vi "boolean mechanical action tests.vi"() -> ()   [LabVIEW 2021, in "Test VIs.lvclass"]
uses:
  Main VIs/Test VIs/Test VIs.lvclass
panel:
  out "Radio Buttons 2":enum32{"Radio Selection 1", "Radio Selection 2"}(radio)
  in  "Radio Buttons":enum32{"Radio Selection 1", "Radio Selection 2"}(radio)
  in  "stop":bool
  out "Boolean 3":bool
  out "Boolean 2":bool
  out "Boolean":bool
  out "Latch Until Released":string
  out "Latch When Released":string
  out "Latch When Pressed":string
  out "Switch Until Released":string
  out "Switch When Released":string
  out "Switch When Pressed":string
  in  "Latch Until Released":bool
  in  "Latch When Released":bool
  in  "Latch When Pressed":bool
  in  "Switch Until Released":bool
  in  "Switch When Released":bool
  in  "Switch When Pressed":bool
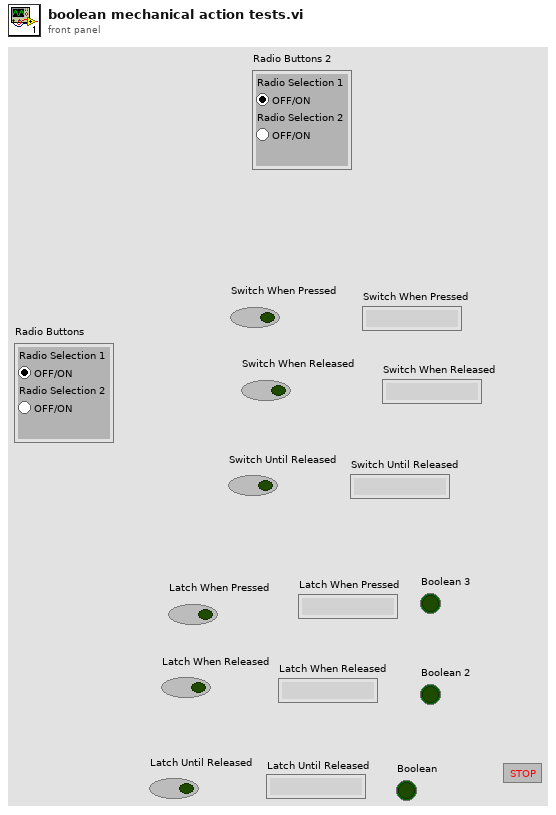
[diagram p1: front panel]
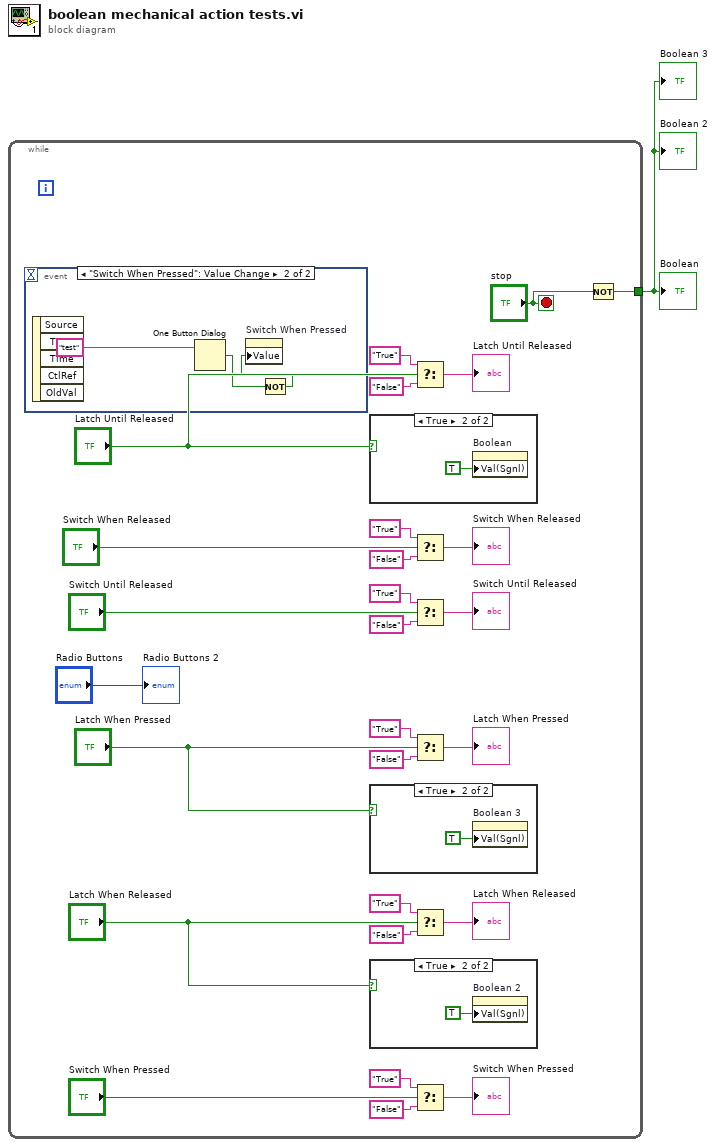
[diagram p0: block diagram]
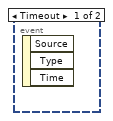
[diagram p2: hidden frame]
diagram:
  n1 = while {
    tunnel: [w4] -> w1
    stop <- "stop" stop-if-true
    n2 = event shown="[1] \"Switch When Pressed\": Value Change" {
      selector: _ -> [_ _]
      dyn-events: _ -> [_ _]
      timeout: _ -> [_ _]
      event Timeout {
        n3 = event-data() -> ()  [unwired: 1 in, 3 out]
      }
      event "Switch When Pressed": Value Change {
        n4 = event-data() -> ()  [unwired: 1 in, 5 out]
        n5 = One Button Dialog(message="test") -> (true=w30:bool)  [unwired: 1 in]
        n6 = Not(x=w30) -> (.not. x?=w29:bool)
        n7 = property on="Switch When Pressed" class="Bool (strict)"("Value"=w29) -> ()  [unwired: 2 in, 2 out]
      }
    }
    n8 = case shown="True" "Latch Until Released" {
      frame False {
      }
      frame True {
        n9 = property on="Boolean" class="Bool (strict)"("Val(Sgnl)"=TRUE ("Value (Signaling)")) -> ()  [unwired: 2 in, 2 out]
      }
    }
    n10 = case shown="True" "Latch When Pressed" {
      frame False {
      }
      frame True {
        n11 = property on="Boolean 3" class="Bool (strict)"("Val(Sgnl)"=TRUE ("Value (Signaling)")) -> ()  [unwired: 2 in, 2 out]
      }
    }
    n12 = case shown="True" "Latch When Released" {
      frame False {
      }
      frame True {
        n13 = property on="Boolean 2" class="Bool (strict)"("Val(Sgnl)"=TRUE ("Value (Signaling)")) -> ()  [unwired: 2 in, 2 out]
      }
    }
    n14 = Select(t="True", s="Latch Until Released", f="False") -> (s? t:f=→"Latch Until Released":string)
    n15 = Select(t="True", s="Switch When Released", f="False") -> (s? t:f=→"Switch When Released":string)
    n16 = Select(t="True", s="Switch Until Released", f="False") -> (s? t:f=→"Switch Until Released":string)
    n17 = Select(t="True", s="Latch When Pressed", f="False") -> (s? t:f=→"Latch When Pressed":string)
    n18 = Select(t="True", s="Latch When Released", f="False") -> (s? t:f=→"Latch When Released":string)
    n19 = Select(t="True", s="Switch When Pressed", f="False") -> (s? t:f=→"Switch When Pressed":string)
    n20 = Not(x="stop") -> (.not. x?=w4:bool)
    "Radio Buttons 2" <- "Radio Buttons"
  }
  "Boolean" <- w1
  "Boolean 2" <- w1
  "Boolean 3" <- w1
